vi "decorateImage.vi"(4 "reticleColor":u32(colorbox)=6618880, 5 "errorIn":errorcluster, 6 "imageRows":i32, 7 "FitCol":i32, 8 "ImageDest":T1, 9 "FitRow":i32, 10 "imageCols":i32, 11 "image":T1) -> (0 "error out":errorcluster, 3 "imageDecorated":T1)   [LabVIEW 2021]
uses:
  <vilib>/vision/Image Controls.llb/IMAQ Image.ctl
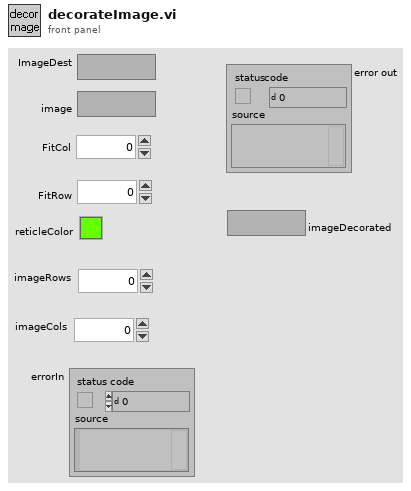
[diagram p1: front panel]
types:
  T1 = typedef "IMAQ Image.ctl" = refnum<image>
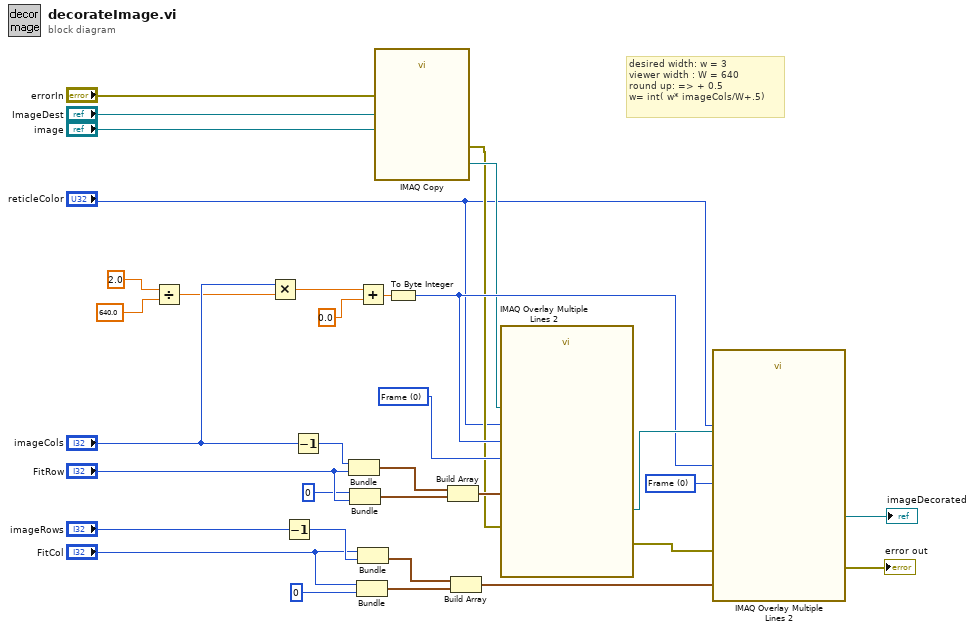
[diagram p0: block diagram]
diagram:
  w25 = u32 0 items=["Frame", "Fill"] ("Drawing Mode (Frame)")
  w24 = u32 0 items=["Frame", "Fill"] ("Drawing Mode (Frame)")
  # "desired width: w = 3\nviewer width : W = 640\nround up: => + 0.5\nw= int( w* imageCols/W+.5)"
  n1 = Divide(x=2.0, y=640.0) -> (x/y=w1:dbl)
  n2 = Multiply(x="imageCols", y=w1) -> (x*y=w16:dbl)
  n3 = Decrement(x="imageRows") -> (x-1=w33:i32)
  n4 = Decrement(x="imageCols") -> (x-1=w31:i32)
  n5 = Bundle(w31, "FitRow"="FitRow") -> (w32:cluster{i32, "FitRow":i32})  [unwired: 1 in]
  n6 = Bundle("element"=0, "FitRow"="FitRow") -> (w22:cluster{"element":i32, "FitRow":i32})  [unwired: 1 in]
  n7 = Bundle("FitCol"="FitCol", "element"=0) -> (w28:cluster{"FitCol":i32, "element":i32})  [unwired: 1 in]
  n8 = Add(x=w16, y=0.0) -> (x+y=w14:dbl)
  n9 = Bundle("FitCol"="FitCol", w33) -> (w27:cluster{"FitCol":i32, i32})  [unwired: 1 in]
  n10 = call "IMAQ Copy"("error in (no error)"="errorIn", "Image Dst"="ImageDest", "Image Src"="image") -> ("error out"=w8:errorcluster, "Image Dst Out"=w11:T1)  [unwired: 3 in]
  n11 = To Byte Integer(number=w14) -> (8bit integer=w13:i8)
  n12 = Build Array(w32, w22) -> (w23:cluster{"element":i32, "FitRow":i32}[])
  n13 = Build Array(w27, w28) -> (w29:cluster{"FitCol":i32, "element":i32}[])
  n14 = call "IMAQ Overlay Multiple Lines 2"("Image"=w11, "Line End Points"=w23, "Drawing Mode (Frame)"=w24, "Color"="reticleColor", "error in (no error)"=w8, "Width"=w13) -> ("Image Out"=w26:T1, "error out"=w7:errorcluster)  [unwired: 8 in]
  n15 = call "IMAQ Overlay Multiple Lines 2"("Image"=w26, "Line End Points"=w29, "Drawing Mode (Frame)"=w25, "Color"="reticleColor", "error in (no error)"=w7, "Width"=w13) -> ("Image Out"=→"imageDecorated":T1, "error out"=→"error out":errorcluster)  [unwired: 8 in]
